vi "Photon_PH.vi"(1 "channel":u16=1, 2 "dtime":u16, 3 "numsync":u16) -> (0 "Event":u32)   [LabVIEW 2012]
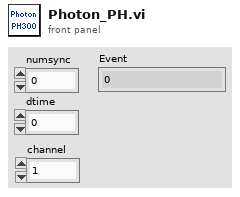
[diagram p1: front panel]
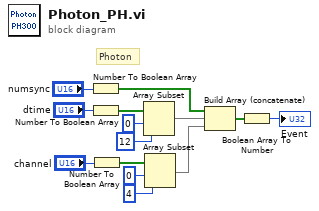
[diagram p0: block diagram]
diagram:
  # "Photon"
  n1 = Number To Boolean Array(number="numsync") -> (Boolean array=w1:bool[])
  n2 = Number To Boolean Array(number="dtime") -> (Boolean array=w11:bool[])
  n3 = Number To Boolean Array(number="channel") -> (Boolean array=w8:bool[])
  n4 = Array Subset(array=w11, index=0, length=12) -> (w5:bool[])
  n5 = Array Subset(array=w8, index=0, length=4) -> (w2:bool[])
  n6 = Build Array (concatenate)(w1, w5, w2) -> (w3:bool[])
  n7 = Boolean Array To Number(Boolean array=w3) -> (number=→"Event":u32)
